vi "OrderSensors.vi"(1 "IR Sensors":T1(array[cluster])) -> (0 "spyder":cluster{"magnitude":dbl, "phase":dbl}[](array[cluster]) {"phase" format="%0.2f"; "magnitude" format="%0.2f"})   [LabVIEW 2014]
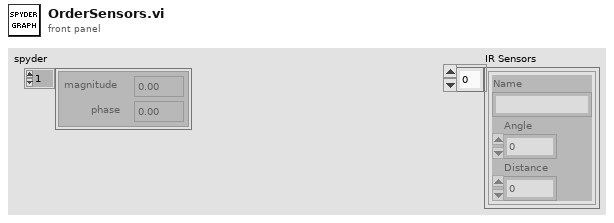
[diagram p1: front panel]
types:
  T1 = cluster{"Name":string, "Angle":dbl, "Distance":dbl}[]
  T2 = cluster{"Name":string, "Angle":dbl, "Distance":dbl}
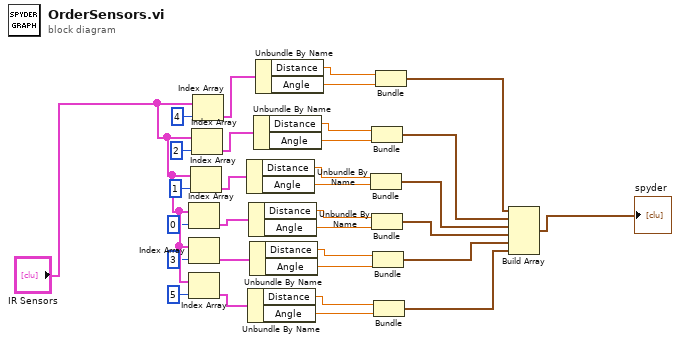
[diagram p0: block diagram]
diagram:
  n1 = Index Array(array="IR Sensors", index=0) -> (element=w22:T2)
  n2 = Index Array(array="IR Sensors", index=3) -> (element=w21:T2)
  n3 = Index Array(array="IR Sensors", index=5) -> (element=w20:T2)
  n4 = Index Array(array="IR Sensors", index=1) -> (element=w23:T2)
  n5 = Index Array(array="IR Sensors", index=2) -> (element=w24:T2)
  n6 = Index Array(array="IR Sensors", index=4) -> (element=w25:T2)
  n7 = Unbundle By Name(w23) -> ("Distance"=w15:dbl, "Angle"=w14:dbl)
  n8 = Unbundle By Name(w20) -> ("Distance"=w9:dbl, "Angle"=w8:dbl)
  n9 = Unbundle By Name(w22) -> ("Distance"=w13:dbl, "Angle"=w12:dbl)
  n10 = Unbundle By Name(w21) -> ("Distance"=w11:dbl, "Angle"=w10:dbl)
  n11 = Unbundle By Name(w24) -> ("Distance"=w17:dbl, "Angle"=w16:dbl)
  n12 = Unbundle By Name(w25) -> ("Distance"=w19:dbl, "Angle"=w18:dbl)
  n13 = Bundle("Distance"=w15, "Angle"=w14) -> (w5:cluster{"Distance":dbl, "Angle":dbl})  [unwired: 1 in]
  n14 = Bundle("Distance"=w17, "Angle"=w16) -> (w6:cluster{"Distance":dbl, "Angle":dbl})  [unwired: 1 in]
  n15 = Bundle("Distance"=w13, "Angle"=w12) -> (w4:cluster{"Distance":dbl, "Angle":dbl})  [unwired: 1 in]
  n16 = Bundle("Distance"=w11, "Angle"=w10) -> (w3:cluster{"Distance":dbl, "Angle":dbl})  [unwired: 1 in]
  n17 = Bundle("Distance"=w9, "Angle"=w8) -> (w2:cluster{"Distance":dbl, "Angle":dbl})  [unwired: 1 in]
  n18 = Bundle("Distance"=w19, "Angle"=w18) -> (w7:cluster{"Distance":dbl, "Angle":dbl})  [unwired: 1 in]
  n19 = Build Array(w7, w6, w5, w4, w3, w2) -> (→"spyder":cluster{"Distance":dbl, "Angle":dbl}[])
